vi "KM_HFLI_get_one_data_point.vi"(0 "Handle In":T1 {"Handle" format="0x%08x"; "Conn" format="0x%08x"}, 2 "Freq Sequence In":dbl[](array[numeric]) format="%#_6p", 5 "Error In":errorcluster, 6 "Harmonic (1=fundamental)":i32=1 min=1 max=66000, 7 "Oscillator (0)":u16, 8 "Order (4)":i32(ring)=4 items=["6, 1st"=1, "12, 2nd"=2, "18, 3rd"=3, "24, 4th"=4, "30, 5th"=5, "36, 6th"=6, "42, 7th"=7, "48, 8th"=8], 9 "Input Demods (0)":u16[](array[numeric])=[0], 10 "Averaging":u16(ring)=1 caption="Averaging (1)" items=["1"=1, "2"=2, "4"=4, "8"=8, "16"=16, "32"=32, "64"=64, "128"=128], 11 "Output Demod (0)":u16, 13 "Signal Output (0)":u16 max=1) -> (14 "Handle Out":T1 {"Handle" format="0x%08x"; "Conn" format="0x%08x"}, 15 "total":dbl, 16 "first":dbl, 17 "Frequency OUT":dbl caption="Frequency (Hz)" format="%_7p", 18 "z OUT":cdb[](array[numeric]), 19 "Error Out":errorcluster)   [LabVIEW 2016]
uses:
  <instrlib>/Zurich Instruments LabOne/Public/ziTypeHandle.ctl
  <instrlib>/Zurich Instruments LabOne/Public/Utility/ziTicksToS_single.vi
  <instrlib>/Zurich Instruments LabOne/Zurich Instruments LabOne.lvlib
panel:
  out "Bandwidth_indic":dbl=100.0 caption="Bandwidth (Hz)" format="%_3p"
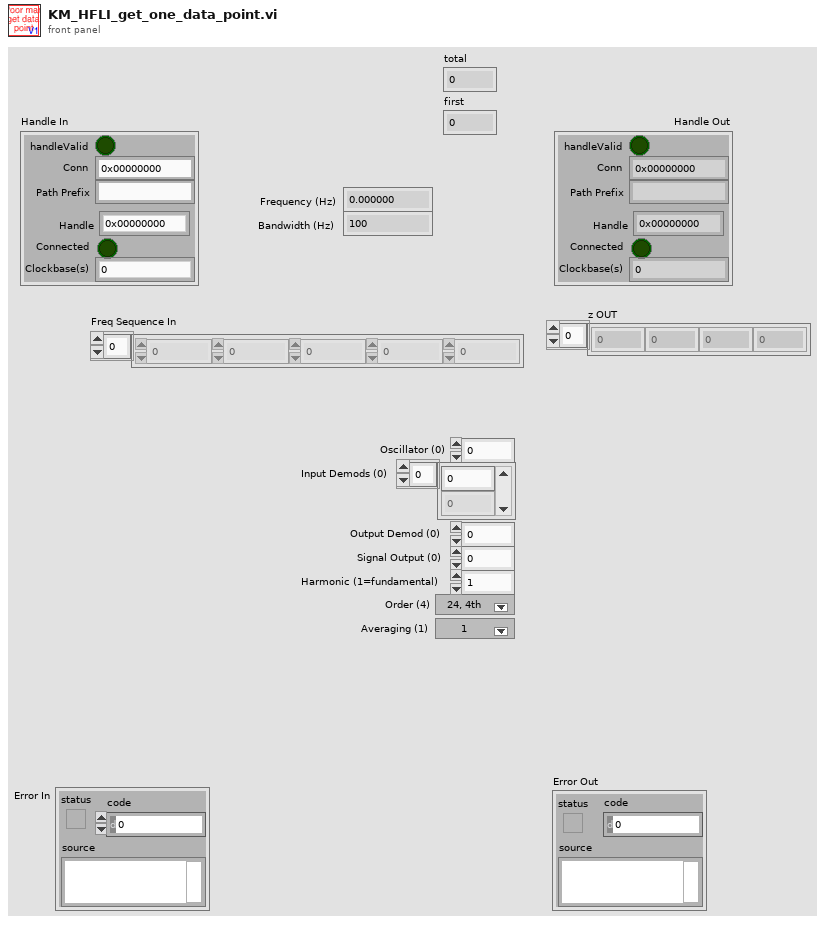
[diagram p1: front panel]
types:
  T1 = typedef "Zurich Instruments LabOne.lvlib/ziTypeHandle.ctl" = cluster{"handleValid":bool, "Conn":u64, "Path Prefix":string, "Handle":u64, "Connected":bool, "Clockbase(s)":dbl}
  T2 = cluster{"Timestamps (ticks)":u64, "X (Vrms)":dbl, "Y (Vrms)":dbl, "Osc Phase (deg)":dbl, "Freq (Hz)":dbl, "DIO":u32, "AuxIn0 (V)":dbl, "AuxIn1 (V)":dbl}
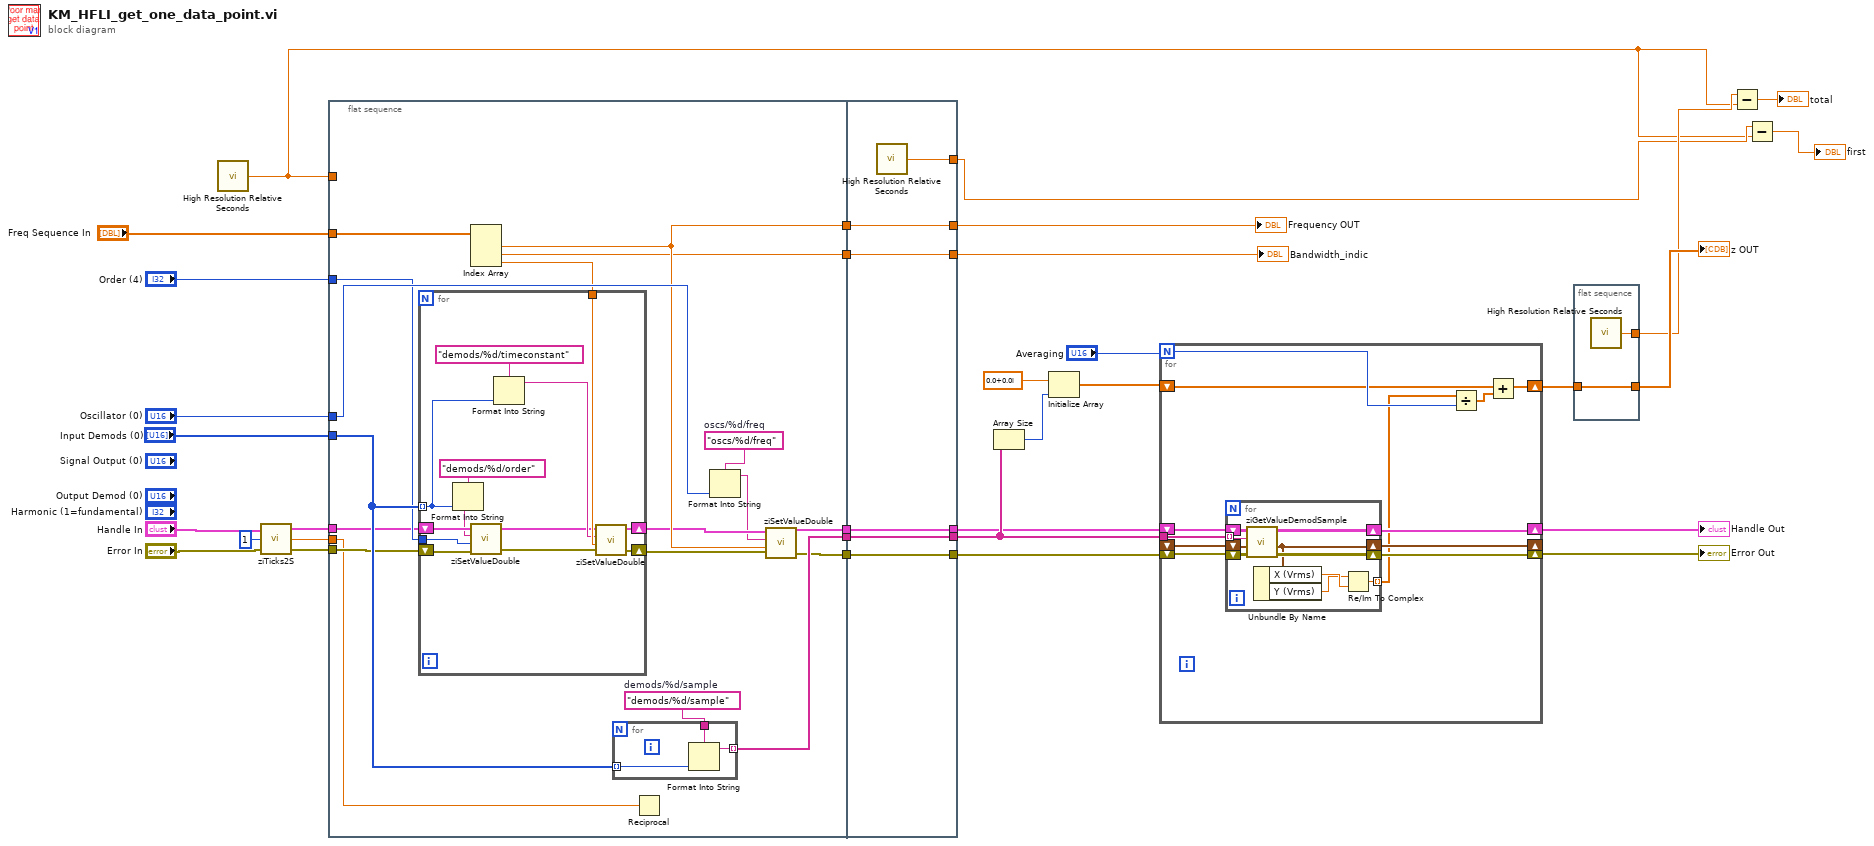
[diagram p0: block diagram]
diagram:
  n1 = call <vilib>:"High Resolution Relative Seconds.vi"() -> ("relative seconds"=w5:dbl)
  n2 = call-poly <instrlib>:"ziTicks2S.vi"("Error In"="Error In", "Timestamp(ticks)"=u64 1, "Handle In"="Handle In") -> ("Error Out"=w22:errorcluster, "Timestamp(s)"=w20:dbl, "Handle Out"=w21:T1)
  n3 = flat-sequence {
    tunnel: "Oscillator (0)" -> [w51]
    tunnel: "Input Demods (0)" -> [w50]
    tunnel: "Order (4)" -> [w49]
    tunnel: "Freq Sequence In" -> [w48]
    tunnel: w22 -> [w40]
    tunnel: w21 -> [w39]
    tunnel: w20 -> [w38]
    tunnel: w5 -> [_]
    tunnel: [w47] -> w13
    tunnel: [w37] -> w12
    tunnel: [w36] -> w11
    tunnel: [w35] -> w10
    tunnel: [w34] -> w1
    tunnel: [w70] -> w14
    tunnel: [w71] -> w15
    tunnel: [w72] -> w19
    tunnel: [w73] -> w25
    tunnel: w13 -> [w73]
    tunnel: w12 -> [w72]
    tunnel: w11 -> [w71]
    tunnel: w10 -> [w70]
    tunnel: [w69] -> w6
    tunnel: [w68] -> w2
    tunnel: w1 -> [w68]
    frame #0 {
      w44 = "oscs/%d/freq"  # oscs/%d/freq
      w46 = "demods/%d/sample"  # demods/%d/sample
      n4 = Index Array(array=w48) -> (element #1=w47:dbl, element #2=w34:dbl, element #3=w45:dbl)  [unwired: 3 in]
      n5 = for {
        tunnel: w50 -> [w52] mode=indexing
        tunnel: w45 -> [w64]
        shift-right: [w61] -> w43
        shift-left: w39 -> [w57]
        shift-right: [w60] -> w42
        shift-left: w40 -> [w58]
        tunnel: w49 -> [w55]
        n6 = Format Into String(format string="demods/%d/order", w52) -> (resulting string=w53:string)  [unwired: 2 in, 1 out]
        n7 = call <instrlib>:"ziSetValueDouble.vi"("Error In"=w58, "Value"=w55, "Path"=w53, "Handle In"=w57) -> ("Error Out"=w59:errorcluster, "Handle Out"=w56:T1)  [unwired: 1 in]
        n8 = Format Into String(format string="demods/%d/timeconstant", w52) -> (resulting string=w62:string)  [unwired: 2 in, 1 out]
        n9 = call <instrlib>:"ziSetValueDouble.vi"("Error In"=w59, "Value"=w64, "Path"=w62, "Handle In"=w56) -> ("Error Out"=w60:errorcluster, "Handle Out"=w61:T1)  [unwired: 1 in]
      }
      n10 = for {
        tunnel: w46 -> [w67]
        tunnel: w50 -> [w66] mode=indexing
        tunnel: [w65] -> w37 mode=indexing
        n11 = Format Into String(format string=w67, w66) -> (resulting string=w65:string)  [unwired: 2 in, 1 out]
      }
      n12 = Reciprocal(x=w38) -> ()  [unwired: 1 out]
      n13 = Format Into String(format string=w44, w51) -> (resulting string=w41:string)  [unwired: 2 in, 1 out]
      n14 = call <instrlib>:"ziSetValueDouble.vi"("Error In"=w42, "Value"=w47, "Path"=w41, "Handle In"=w43) -> ("Error Out"=w36:errorcluster, "Handle Out"=w35:T1)  [unwired: 1 in]
    }
    frame #1 {
      n15 = call <vilib>:"High Resolution Relative Seconds.vi"() -> ("relative seconds"=w69:dbl)
    }
  }
  n16 = Array Size(array=w19) -> (size(s)=w18:i32)
  n17 = Initialize Array(cdb 0.0+0.0i ("element"), w18) -> (w16:cdb[])
  n18 = for {
    N: "Averaging" -> [w80]
    shift-right: [w85] -> w33
    shift-left: w14 -> [w79]
    shift-right: [w84] -> w32
    shift-left: w15 -> [w77]
    tunnel: w19 -> [w83]
    shift-right: [w82] -> _
    shift-left: _ -> [w78]
    shift-right: [w74] -> w9
    shift-left: w16 -> [w75]
    n19 = for {
      shift-right: [w93] -> w84
      shift-left: w77 -> [w94]
      shift-right: [w92] -> w85
      shift-left: w79 -> [w95]
      shift-right: [w90] -> w82
      shift-left: w78 -> [w91]
      tunnel: w83 -> [w89] mode=indexing
      tunnel: [w88] -> w76 mode=indexing
      n20 = call <instrlib>:"ziGetValueDemodSample.vi"("error in"=w94, "Demod Sample In"=w91, "Path"=w89, "Handle In"=w95) -> ("error out"=w93:errorcluster, "Demod Sample Out"=w90:T2, "Handle Out"=w92:T1)  [unwired: 1 in]
      n21 = Unbundle By Name(w90) -> ("X (Vrms)"=w87:dbl, "Y (Vrms)"=w86:dbl)
      n22 = Re/Im To Complex(1:w87, 2:w86) -> (0:w88:cdb)
    }
    n23 = Divide(x=w76, y=w80) -> (x/y=w81:cdb[])
    n24 = Add(x=w75, y=w81) -> (x+y=w74:cdb[])
  }
  "Handle Out" <- w33
  "Error Out" <- w32
  n25 = flat-sequence {
    tunnel: [w97] -> w8
    tunnel: w9 -> [w97]
    tunnel: [w96] -> w7
    frame #0 {
      n26 = call <vilib>:"High Resolution Relative Seconds.vi"() -> ("relative seconds"=w96:dbl)
    }
  }
  n27 = Subtract(x=w7, y=w5) -> (x-y=→"total":dbl)
  n28 = Subtract(x=w6, y=w5) -> (x-y=→"first":dbl)
  "Frequency OUT" <- w25
  "z OUT" <- w8
  "Bandwidth_indic" <- w2
